vi "Build Device Combo List.vi"(7 "Previous Value":string, 11 "Devices":refnum<class "Device.lvclass">[](array[class])) -> (2 "Value":string, 3 "Strings":string[](array[string]))   [LabVIEW 2020, in "PicoG-App.lvlib" / "AppDetailPanel.lvclass"]
uses:
  AppDetailPanel.lvclass
  Device/Device.lvclass
  Builds/picoG/ppl/PicoG-Core.lvlibp/PicoG-Processor/PicoG-Core/Resource/Resource.lvclass
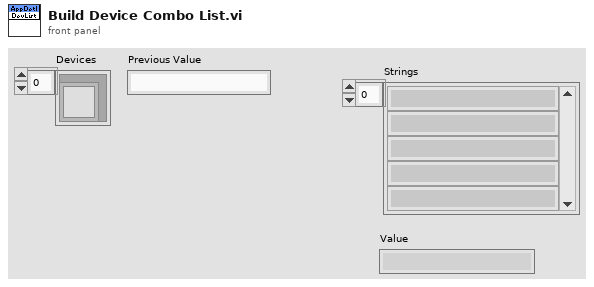
[diagram p1: front panel]
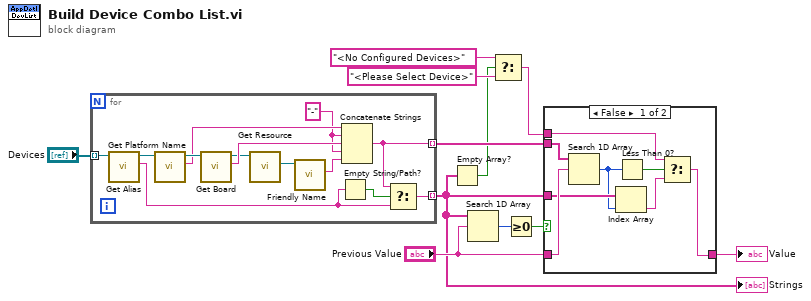
[diagram p0: block diagram]
diagram:
  n1 = for {
    tunnel: "Devices" -> [w24] mode=indexing
    tunnel: [w18] -> w7 mode=indexing
    tunnel: [w15] -> w5 mode=indexing
    w19 = "-" ("string")
    n2 = call "Get Alias.vi"("Device in"=w24) -> ("Alias"=w16:string, "Device out"=w23:refnum<class "Device.lvclass">)  [unwired: 8 in, 1 out]
    n3 = call "Get Platform Name.vi"("Device in"=w23) -> ("Platform"=w20:string, "Device out"=w22:refnum<class "Device.lvclass">)  [unwired: 8 in, 1 out]
    n4 = call "Get Board.vi"("Device in"=w22) -> ("Board"=w21:string, "Device out"=w14:refnum<class "Device.lvclass">)  [unwired: 8 in, 1 out]
    n5 = call "Get Resource.vi"("Device in"=w14) -> ("Resource"=w13:refnum<class "Resource.lvclass">)  [unwired: 8 in, 2 out]
    n6 = call-dynamic "Friendly Name.vi"("DeployResource in"=w13) -> ("Friendly Name"=w12:string)  [unwired: 8 in, 2 out]
    n7 = Empty String/Path?(string/path=w16) -> (empty?=w17:bool)
    n8 = Concatenate Strings(w20, w19, w21, w19, w12) -> (w18:string)
    n9 = Select(t=w18, s=w17, f=w16) -> (s? t:f=w15:string)
  }
  "Strings" <- w5
  n10 = Empty Array?(array=w5) -> (empty?=w2:bool)
  n11 = Search 1D Array(1D array=w5, element="Previous Value") -> (index of element=w10:i32)  [unwired: 1 in]
  n12 = Select(t="<No Configured Devices>", s=w2, f="<Please Select Device>") -> (s? t:f=w1:string)
  n13 = Greater Or Equal To 0?(x=w10) -> (x >= 0?=w9:bool)
  n14 = case shown="False" w9 {
    tunnel: "Previous Value" -> [w31 w33]
    tunnel: w5 -> [w30 _]
    tunnel: w7 -> [w32 _]
    tunnel: [w26 w33] -> w6
    tunnel: w1 -> [w25 _]
    frame False {
      n15 = Search 1D Array(1D array=w32, element=w31) -> (index of element=w29:i32)  [unwired: 1 in]
      n16 = Index Array(array=w30, index=w29) -> (element=w27:string)
      n17 = Less Than 0?(x=w29) -> (x < 0?=w28:bool)
      n18 = Select(t=w25, s=w28, f=w27) -> (s? t:f=w26:string)
    }
    frame True {
    }
  }
  "Value" <- w6
